vi "Read shift.vi"(11 "Node in":refnum<class "Node.lvclass">) -> (2 "shift":i64, 3 "Node out":refnum<class "Node.lvclass">)   [LabVIEW 2023, in "d20.lvlib" / "Node.lvclass"]
uses:
  Node.lvclass
  Node.lvclass/Node.ctl
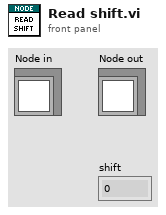
[diagram p1: front panel]
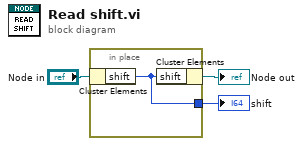
[diagram p0: block diagram]
diagram:
  n1 = in-place {
    in-place-border: [w4] -> w1
    n2 = in-place-cluster #1("Node in") -> ("shift"=w4:i64)
    n3 = in-place-cluster #1("shift"=w4) -> (→"Node out":refnum<class "Node.lvclass">)
  }
  "shift" <- w1
